vi "例程22-二进制文件的读取.vi"() -> ()   [LabVIEW 2016]
panel:
  out "数据":dbl[](array[numeric])
  out "读出的数据":dbl[](graph)
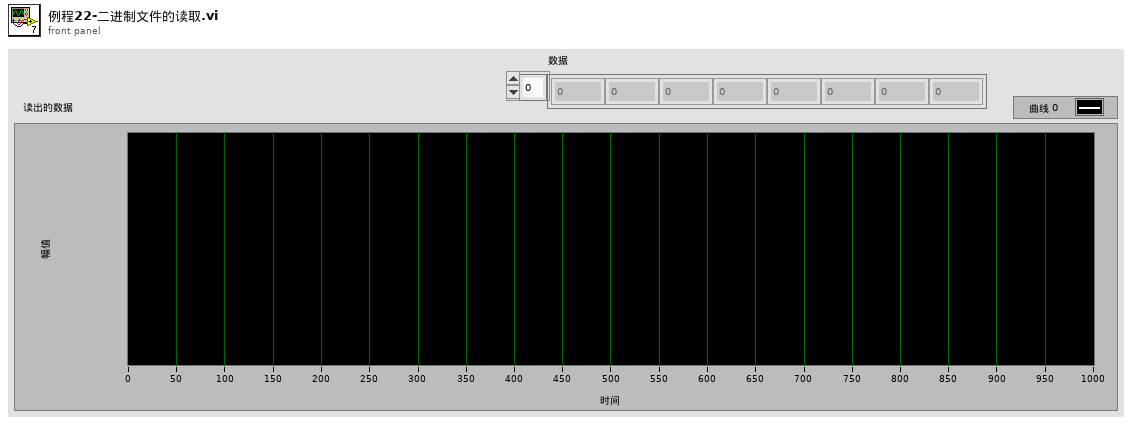
[diagram p1: front panel]
types:
  T1 = enum16{"big-endian, network order", "native, host order", "little-endian"}
  T2 = enum16{"deny read/write", "deny write-only", "deny none"}
  T3 = enum16{"open", "replace", "create", "open or create", "replace or create", "replace or create with confirmation"}
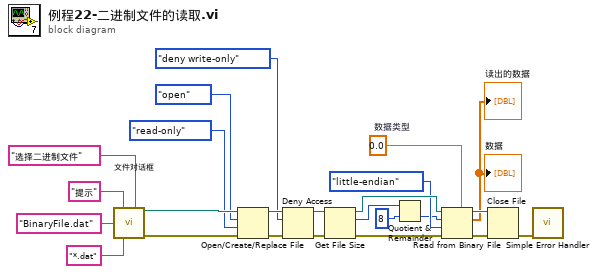
[diagram p0: block diagram]
diagram:
  w2 = 0.0  # 数据类型
  n1 = call "文件对话框"("prompt"="提示", "button label"="选择二进制文件", "default name"="BinaryFile.dat", "pattern (all files)"="*.dat") -> ("selected path"=w23:path, "error out"=w10:errorcluster)  [unwired: 8 in, 2 out]
  n2 = Open/Create/Replace File(file path (use dialog)=w23, error in=w10, operation (0:open)=T3."open" ("操作(0:open)"), access (0:read/write)=enum16{"read/write", "read-only", "write-only"}."read-only" ("权限(0:read/write)")) -> (refnum out=w17:refnum<file>, error out=w18:errorcluster)  [unwired: 2 in, 1 out]
  n3 = Deny Access(4:w18, 6:T2."deny write-only" ("限制模式(0:读/写限制)"), 7:w17) -> (0:w15:errorcluster, 3:w11:refnum<file>)
  n4 = Get File Size(file=w11, error in=w15) -> (refnum out=w12:refnum<file>, size (in bytes)=w6:i64, 0:w14:errorcluster)
  n5 = Quotient & Remainder(x=w6, y=i64 8) -> (floor(x/y)=w3:i64)  [unwired: 1 out]
  n6 = Read from Binary File(5:w2, 8:w14, 9:T1."little-endian" ("字节顺序(0:big-endian, network order)"), 10:w3, 11:w12) -> (0:w13:errorcluster, 2:→"读出的数据" →"数据":dbl[], 3:w16:refnum<file>)  [unwired: 1 in, 1 out]
  n7 = Close File(refnum=w16, error in=w13) -> (error out=w19:errorcluster)  [unwired: 1 out]
  n8 = call <vilib>:"Simple Error Handler.vi"("error in (no error)"=w19) -> ()  [unwired: 4 in, 5 out]
